vi "Read Multi Data.vi"(8 "error in (no error)":errorcluster, 11 "Multi Data in":refnum<class "Multi Data.lvclass">) -> (0 "error out":errorcluster, 1 "Data Alias Array":string[](array[string]), 2 "Data Array":refnum<class "Data.lvclass">[](array[class]), 3 "Multi Data out":refnum<class "Multi Data.lvclass">, 5 "Alias":string)   [LabVIEW 2020, in "Publisher.lvlib" / "Multi Data.lvclass"]
doc: "Read the class data."
uses:
  Multi Data.lvclass
  PPL/HDH.Data.Generic.lvlibp/Data.lvclass
  Multi Data.lvclass/Multi Data.ctl
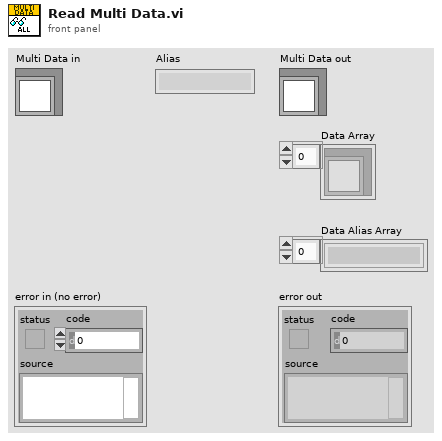
[diagram p1: front panel]
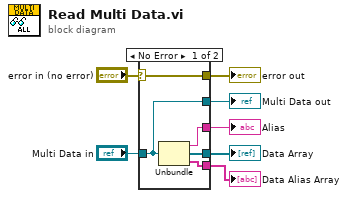
[diagram p0: block diagram]
diagram:
  n1 = case shown="No Error" "error in (no error)" {
    selector: "error in (no error)" -> [w12 w13]
    tunnel: [w12 w13] -> w6
    tunnel: [w8 w14] -> w4
    tunnel: "Multi Data in" -> [w8 w14]
    tunnel: [w11 _] -> w3
    tunnel: [w10 _] -> w2
    tunnel: [w9 _] -> w1
    frame No Error {
      n2 = Unbundle(w8) -> (w11:string, w10:refnum<class "Data.lvclass">[], w9:string[])
    }
    frame Error {
    }
  }
  "error out" <- w6
  "Multi Data out" <- w4
  "Alias" <- w3
  "Data Array" <- w2
  "Data Alias Array" <- w1
